vi "EventCreate.vi"(8 "error in (no error)":errorcluster, 11 "Execute":refnum<class "Execute.lvclass">) -> (0 "error out":errorcluster, 3 "Execute":refnum<class "Execute.lvclass">)   [LabVIEW 2018, in "QMH_Class.lvlib" / "TestManager.lvlib" / "Execute.lvclass"]
uses:
  Execute.lvclass
  Execute.lvclass/Execute.ctl
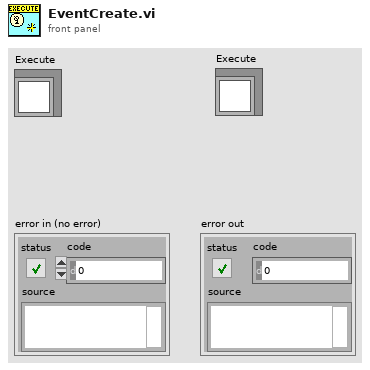
[diagram p1: front panel]
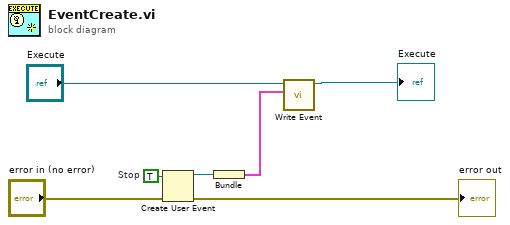
[diagram p0: block diagram]
diagram:
  w5 = TRUE  # Stop
  n1 = Create User Event(user event datatype=w5, error in="error in (no error)") -> (user event=w4:refnum<user-event>, error out=→"error out":errorcluster)
  n2 = Bundle("Stop"=w4) -> (w3:cluster{"Stop":refnum<user-event>})  [unwired: 1 in]
  n3 = call "Write Event.vi"("Event"=w3, "Execute"="Execute") -> ("Execute"=→"Execute":refnum<class "Execute.lvclass">)  [unwired: 8 in, 1 out]
